vi "Wait-for-message.vi"(8 "error in (no error)":errorcluster, 11 "Client in":T1) -> (0 "error out":errorcluster, 1 "New message?":bool, 2 "Message":refnum<class "Message.lvclass">, 3 "Client out":T1)   [LabVIEW 2013, in "Client.lvlib" / "Client.lvclass"]
doc: "Monitors the incomming communication channel (client channel) for new messages.\nThe monitoring will timeout based on the 'Heartbeat interval' parameter in the client settings. The timeout time is 80% of the heartbeat interval value, to allow the client to send a heartbeat message and have it processed by the server. The heartbeat is separate functionality, acessed through the 'Send-heartbeat' function."
uses:
  Client.lvclass
  Object-reference.ctl
  Messages/Sources/Message.lvclass
  Client.lvclass/Client.ctl
  Read Client channel.vi
  Read Heartbeat interval.vi
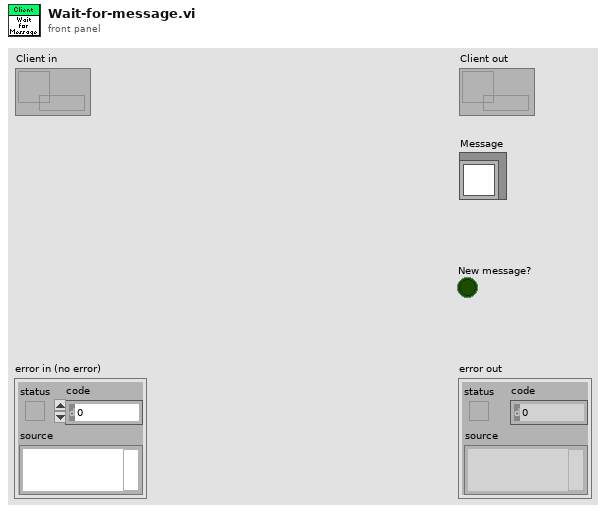
[diagram p1: front panel]
types:
  T1 = typedef "Client.lvlib/Client.lvclass/Object-reference.ctl" = refnum<data-value>
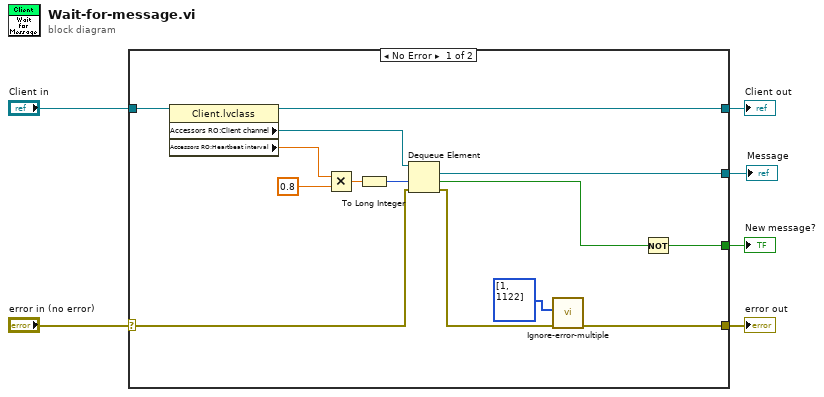
[diagram p0: block diagram]
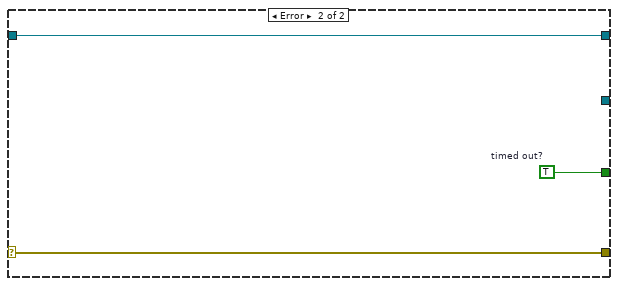
[diagram p2: hidden frame]
diagram:
  n1 = case shown="No Error" "error in (no error)" {
    selector: "error in (no error)" -> [w18 w23]
    tunnel: [w7 w23] -> w5
    tunnel: [w19 w22] -> w3
    tunnel: "Client in" -> [w20 w22]
    tunnel: [w14 w21] -> w2
    tunnel: [w15 _] -> w1
    frame No Error {
      n2 = property class="Client.lvclass"(reference=w20) -> (reference out=w19:T1, "Accessors RO:Client channel"=w17:refnum<queue>, "Accessors RO:Heartbeat interval"=w13:dbl)  [unwired: 1 in, 1 out]
      n3 = Multiply(x=w13, y=0.8) -> (x*y=w12:dbl)
      n4 = To Long Integer(number=w12) -> (32bit integer=w10:i32)
      n5 = Dequeue Element(queue=w17, timeout in ms (-1)=w10, error in (no error)=w18) -> (element=w15:refnum<class "Message.lvclass">, timed out?=w16:bool, error out=w8:errorcluster)  [unwired: 1 out]
      n6 = call "Ignore-error-multiple.vi"("error in (no error)"=w8, "Errors to ignore (1)"=i32[] [1, 1122]) -> ("error out"=w7:errorcluster)  [unwired: 9 in]
      n7 = Not(x=w16) -> (.not. x?=w14:bool)
    }
    frame Error {
      w21 = TRUE  # timed out?
    }
  }
  "error out" <- w5
  "Client out" <- w3
  "New message?" <- w2
  "Message" <- w1
